vi "X Axis Format String Read.vi"(8 "error in (no error)":errorcluster, 11 "3D Plot.lvclass in":refnum<class "3D Plot.lvclass">) -> (0 "error out":errorcluster, 1 "X Axis Format":string, 3 "3D Plot.lvclass out":refnum<class "3D Plot.lvclass">)   [LabVIEW 2020, in "3D Plot.lvclass"]
uses:
  <vilib>/Math Plots/3D Math Plots/3D Plot/3D Plot/3D Plot.lvclass
  <vilib>/Math Plots/3D Math Plots/3D Plot/3D Plot/3D Plot.lvclass/3D Plot.ctl
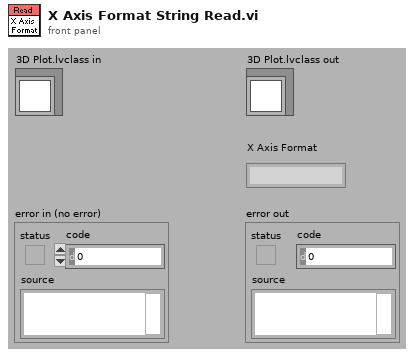
[diagram p1: front panel]
types:
  T1 = typedef "3D Plot.lvclass/Format Property.ctl" = string[]
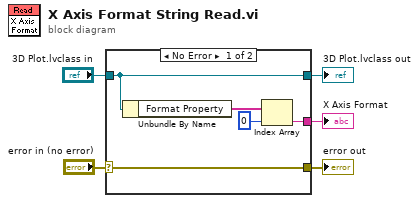
[diagram p0: block diagram]
diagram:
  n1 = case shown="No Error" "error in (no error)" {
    selector: "error in (no error)" -> [w10 w12]
    tunnel: [w7 _] -> w5
    tunnel: "3D Plot.lvclass in" -> [w9 w11]
    tunnel: [w10 w12] -> w2
    tunnel: [w9 w11] -> w1
    frame No Error {
      n2 = Unbundle By Name(w9) -> ("Format Property"=w8:T1)
      n3 = Index Array(array=w8, index=0) -> (element=w7:string)
    }
    frame Error {
    }
  }
  "error out" <- w2
  "X Axis Format" <- w5
  "3D Plot.lvclass out" <- w1
